vi "Read Pinmap.vi"(8 "error in (no error)":errorcluster, 11 "Protocol Interface in":refnum<class "Protocol Interface.lvclass">) -> (0 "error out":errorcluster, 2 "Pinmap":path, 3 "Protocol Interface out":refnum<class "Protocol Interface.lvclass">)   [LabVIEW 2018]
uses:
  Protocol Interface.lvclass
  C:/P4 Workspace/PC Client/Solutions/5g_eap/trunk/1.0/HiSi5GmmWave/Pattern_Gen_Tool/Plugins/SouceCode/Protocol Interface/FPF.lvlibp/Factory Plugin Framework.lvclass
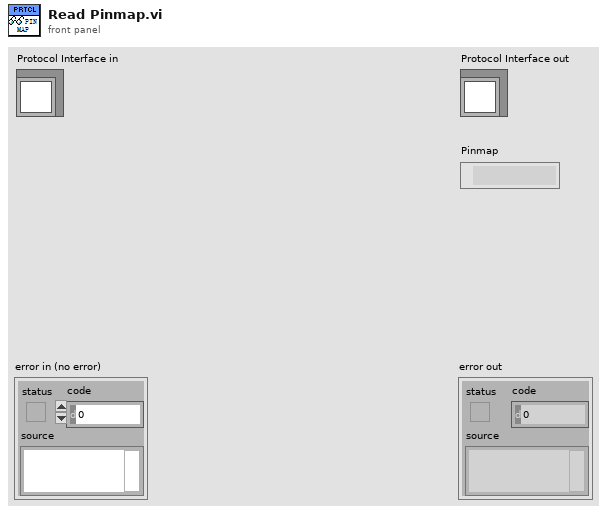
[diagram p1: front panel]
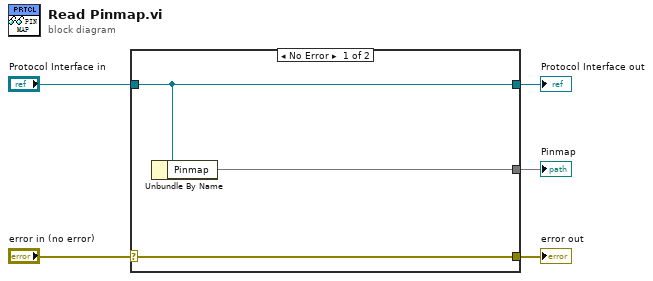
[diagram p0: block diagram]
diagram:
  n1 = case shown="No Error" "error in (no error)" {
    selector: "error in (no error)" -> [w8 w9]
    tunnel: [w8 w9] -> w4
    tunnel: [w7 w10] -> w2
    tunnel: "Protocol Interface in" -> [w7 w10]
    tunnel: [w6 _] -> w1
    frame No Error {
      n2 = Unbundle By Name(w7) -> ("Pinmap"=w6)
    }
    frame Error {
    }
  }
  "error out" <- w4
  "Protocol Interface out" <- w2
  "Pinmap" <- w1
